vi "Tektronix DPO MSO 2000 4000 Series Acquire Digital Voltmeter Example.vi"() -> ()   [LabVIEW 2017]
doc: "This example illustrates how to configure and read a digital voltmeter measurement.\n\n<B>Note:</B>\n(1) This VI is available for MDO3000 Series only.\n\n(2) Requires option MDO3DVM to be installed."
uses:
  <instrlib>/Tektronix DPO MSO 2000 4000 Series/Tektronix DPO MSO 2000 4000 Series.lvlib
panel:
  in  "VISA Resource Name":refnum<visa-resource-name>
  out "Digital Voltmeter Frequency":dbl
  out "Digital Voltmeter Value":dbl
  in  "Source Channel (0: Channel 1)":i32(ring) items=["Channel 1", "Channel 2", "Channel 3", "Channel 4"]
  in  "Digital Voltmeter Type (2: DC)":i32(ring)=2 items=["ACRMS", "ACDCRMS", "DC", "FREQ", "OFF"]
  in  "Auto Range (F: Disable)":bool
  # "(C)2006 - 2016. National Instruments Corporation. ALL RIGHTS RESERVED."
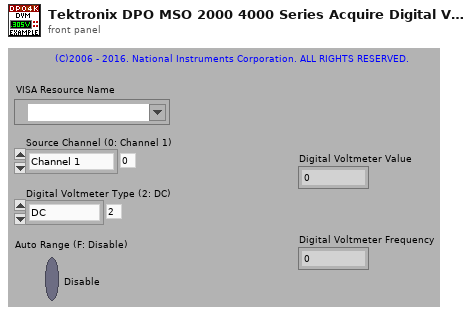
[diagram p1: front panel]
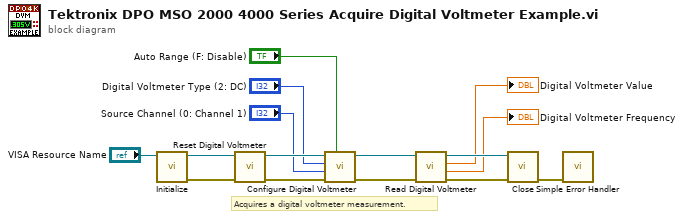
[diagram p0: block diagram]
diagram:
  # "Acquires a digital voltmeter measurement."
  n1 = call <instrlib>:"Initialize.vi"("VISA resource name"="VISA Resource Name") -> ("error out"=w13:errorcluster, "VISA resource name out"=w14:refnum<visa-resource-name>)  [unwired: 9 in]
  n2 = call <instrlib>:"Reset Digital Voltmeter.vi"("error in (no error)"=w13, "VISA resource name"=w14) -> ("error out"=w11:errorcluster, "VISA resource name out"=w12:refnum<visa-resource-name>)  [unwired: 8 in]
  n3 = call <instrlib>:"Configure Digital Voltmeter.vi"("Auto Range (F: Disable)"="Auto Range (F: Disable)", "error in (no error)"=w11, "Source Channel (0: Channel 1)"="Source Channel (0: Channel 1)", "Digital Voltmeter Type (4: OFF)"="Digital Voltmeter Type (2: DC)", "VISA resource name"=w12) -> ("error out"=w9:errorcluster, "VISA resource name out"=w10:refnum<visa-resource-name>)  [unwired: 5 in]
  n4 = call <instrlib>:"Read Digital Voltmeter.vi"("error in (no error)"=w9, "VISA resource name"=w10) -> ("error out"=w4:errorcluster, "Digital Voltmeter Frequency"=→"Digital Voltmeter Frequency":dbl, "Digital Voltmeter Value"=→"Digital Voltmeter Value":dbl, "VISA resource name out"=w5:refnum<visa-resource-name>)  [unwired: 6 in]
  n5 = call <instrlib>:"Close.vi"("error in (no error)"=w4, "VISA resource name"=w5) -> ("error out"=w15:errorcluster)  [unwired: 9 in]
  n6 = call <vilib>:"Simple Error Handler.vi"("error in (no error)"=w15) -> ()  [unwired: 4 in, 5 out]
